vi "LVClass_CorrectionDataManager GetExperienceCommands.vi"(0 "CorrectionDataManager in":refnum<class "CorrectionDataManager.lvclass">, 5 "N° actuator":i32, 11 "error in (no error)":errorcluster) -> (4 "CorrectionDataManager out":refnum<class "CorrectionDataManager.lvclass">, 8 "First DeltaCommand":sgl[](array[numeric]), 10 "Second DeltaCommand":sgl[](array[numeric]), 15 "error out":errorcluster)   [LabVIEW 2020, in "CorrectionDataManager.lvclass"]
doc: "Get experiment command applied for calibration steps count index.\n\n--------------------------------------------------------------------------------\n\n<B>corrdata_managerIn </B> : CorrDataManager object.\n<B>corrdata_managerOut </B> : CorrDataManager object.\n<B>index </B> : Index of the calibration step.\n<B>commands </B> : Wavefront corrector commands associated to the index calibration step.\n<B>ErrorIn </B> : Error\n<B>ErrorOut </B> : Error\n\n--------------------------------------------------------------------------------"
uses:
  CorrectionDataManager.lvclass
  CorrectionDataManager.lvclass/CorrectionDataManager.ctl
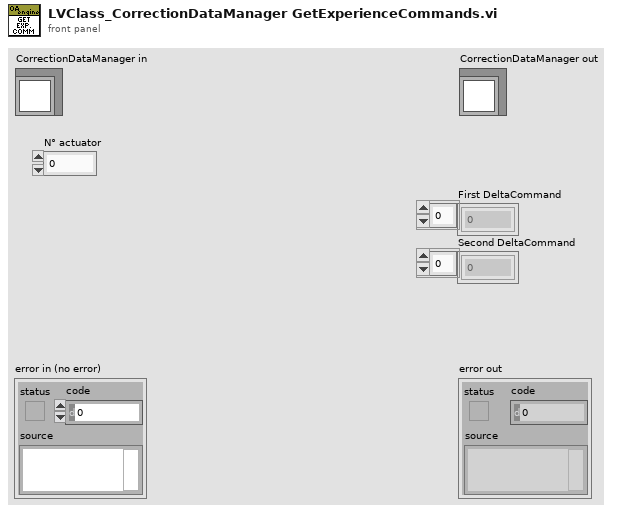
[diagram p1: front panel]
types:
  T1 = typedef "Wavefront Corrector states - ONE.ctl" = cluster{"Max":sgl, "Min":sgl, "Validity":enum16{"valid", "fixed", "invalid"}, "Fixed_Position":sgl}
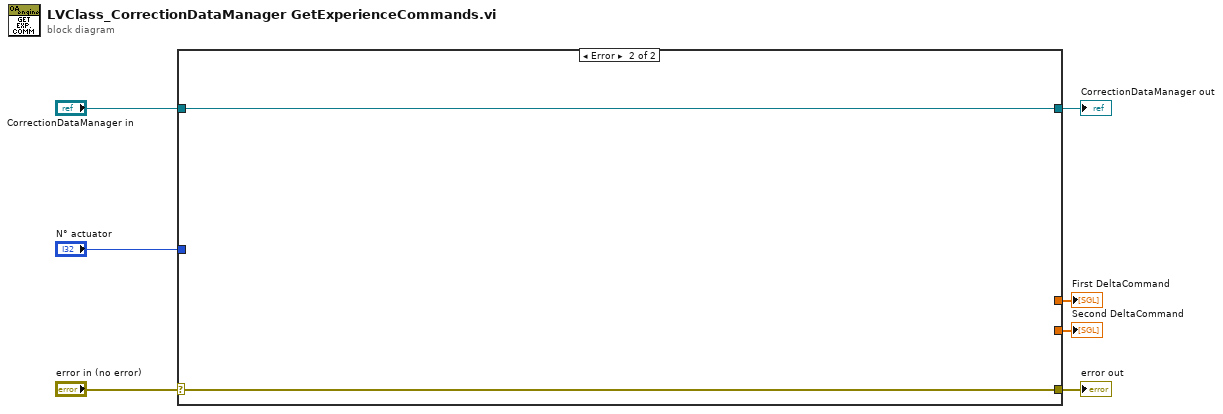
[diagram p0: block diagram]
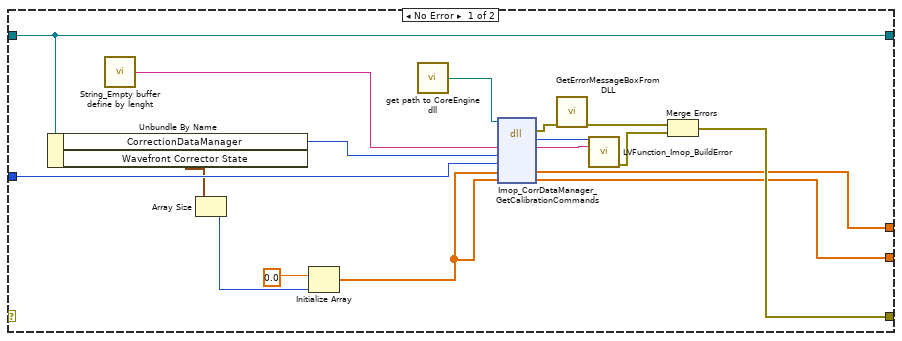
[diagram p2: hidden frame]
diagram:
  n1 = case shown="Error" "error in (no error)" {
    selector: "error in (no error)" -> [_ w26]
    tunnel: [w17 w26] -> w7
    tunnel: [w15 w25] -> w6
    tunnel: "CorrectionDataManager in" -> [w15 w25]
    tunnel: "N° actuator" -> [w14 _]
    tunnel: [w13 _] -> w2
    tunnel: [w12 _] -> w1
    frame No Error {
      n2 = Unbundle By Name(w15) -> ("CorrectionDataManager"=w16:i32, "Wavefront Corrector State"=w11:T1[])
      n3 = call "String_Empty buffer define by lenght.vi"() -> ("Empty buffer"=w22:string)  [unwired: 1 in]
      n4 = Array Size(array=w11) -> (size(s)=w10:i32)
      n5 = Initialize Array(sgl 0.0, w10) -> (w8:sgl[])
      n6 = call "get path to CoreEngine dll.vi"() -> ("path to c_interface_vc100.dll"=w21:path)  [unwired: 12 in, 3 out]
      n7 = dll-call lib="D:/soft/HASO_v3/SVN_trunk/ImOpCoreEngine4_LV2011/DLLs/c_interface_vc100.dll" fn="Imop_CorrDataManager_GetCalibrationCommands"(path in=w21, "message"=w22, "corrdata_manager"=w16, "experience_index"=w14, "First command_push_positive"=w8, "Second command_pull_negative"=w8) -> (error out=w20:errorcluster, "return type"=w24:i32, "message"=w23:string, "First command_push_positive"=w13:sgl[], "Second command_pull_negative"=w12:sgl[])  [unwired: 4 in, 1 out]
      n8 = call "GetErrorMessageBoxFromDLL.vi"("error IN"=w20) -> ("error OUT"=w19:errorcluster)  [unwired: 10 in]
      n9 = call "LVFunction_Imop_BuildError.vi"("code"=w24, "String to Prepend to source (\"\")"=w23) -> ("error out"=w18:errorcluster)  [unwired: 13 in]
      n10 = Merge Errors(w19, w18) -> (w17:errorcluster)
    }
    frame Error {
    }
  }
  "error out" <- w7
  "CorrectionDataManager out" <- w6
  "First DeltaCommand" <- w2
  "Second DeltaCommand" <- w1
